vi "Config File Checker v1.2.vi"(8 "Error In":errorcluster) -> (0 "error out":errorcluster, 2 "All Para":cluster{"Auto Para":T1, "General Para 2":T2}={"Auto Para"={"Agitator Delays"=[250, 600], "TF Delays"=[400, 800, 2, 8000], "Insertion Delays"=[100, 400], "Cutting Delays"=[150, 250, 50], "PF Delays"=[300, 8000], "Measur. Delays"=[200.0, 188.9, 1.0], "Reject Delays"=[500], "BF Delays"=[1000, 1000], "P&P Delays"=[1000]}, "General Para 2"={"Max. Cons."=5.0, "Offset 1"=0.0, "Offset 2"=0.0, "Offset 3"=0.0, "Offset 4"=-0.6, "OutputPause"=500.0, "RejectPause"=500.0, "IndexTimeout"=0.0}} {"General Para 2"."Offset 4" format="%.2f"; "General Para 2"."Offset 3" format="%.2f"; "General Para 2"."Offset 2" format="%.2f"; "General Para 2"."Offset 1" format="%.2f"}, 3 "password":string, 5 "file path out":path)   [LabVIEW 2021]
doc: "v1.2:\n- Created new folder if 'data' folder does not exist\n\nV1.1:\n- changed the location of searching and creating the file"
uses:
  RT/Controls/Auto Delays.ctl
  Controls/General Para.ctl
  HMI/Controls/Logging FGV.ctl
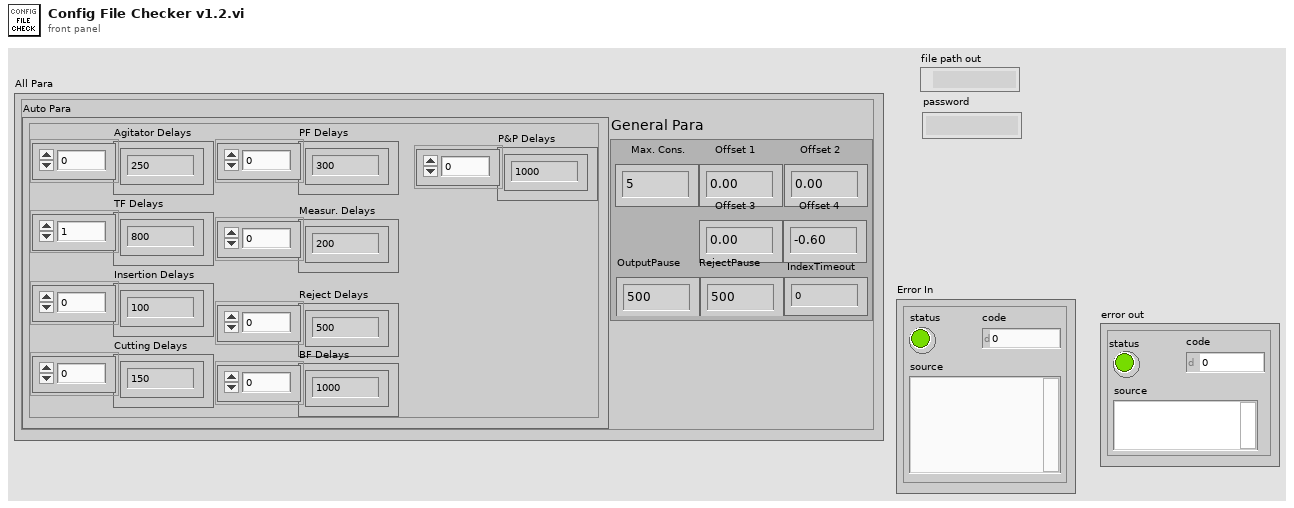
[diagram p1: front panel]
types:
  T1 = typedef "Auto Delays.ctl" = cluster{"Agitator Delays":u32[], "TF Delays":u32[], "Insertion Delays":u32[], "Cutting Delays":u32[], "PF Delays":u32[], "Measur. Delays":dbl[], "Reject Delays":u32[], "BF Delays":u32[], "P&P Delays":u32[]}
  T2 = typedef "General Para.ctl" = cluster{"Max. Cons.":dbl, "Offset 1":dbl, "Offset 2":dbl, "Offset 3":dbl, "Offset 4":dbl, "OutputPause":dbl, "RejectPause":dbl, "IndexTimeout":dbl}
  T3 = typedef "Logging FGV.ctl" = enum16{"Start Shift", "Reload Values", "Log Index", "Read Shift", "Close Shift", "Save Values"}
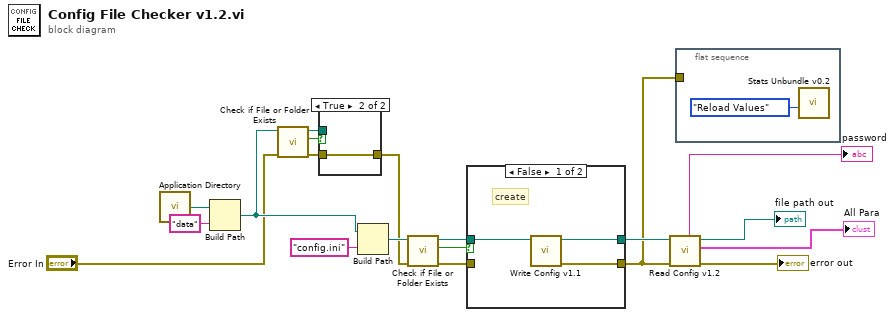
[diagram p0: block diagram]
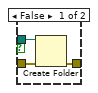
[diagram p2: hidden frame]
diagram:
  n1 = call <vilib>:"Application Directory.vi"() -> ("Application Directory"=w12:path)
  n2 = Build Path(base path=w12, name or relative path="data") -> (appended path=w10:path)
  n3 = call <vilib>:"Check if File or Folder Exists.vi"("error in (no error)"="Error In", "path"=w10) -> ("error out"=w8:errorcluster, "file or folder exists?"=w9:bool, "dup path"=w7:path)  [unwired: 7 in]
  n4 = case shown="True" w9 {
    tunnel: w8 -> [w22 w23]
    tunnel: w7 -> [w21 _]
    tunnel: [w20 w23] -> w5
    frame False {
      n5 = Create Folder(path (use dialog)=w21, error in=w22) -> (error out=w20:errorcluster)  [unwired: 1 in, 2 out]
    }
    frame True {
    }
  }
  n6 = Build Path(base path=w10, name or relative path="config.ini") -> (appended path=w18:path)
  n7 = call <vilib>:"Check if File or Folder Exists.vi"("error in (no error)"=w5, "path"=w18) -> ("error out"=w15:errorcluster, "file or folder exists?"=w17:bool, "dup path"=w16:path)  [unwired: 7 in]
  n8 = case shown="False" w17 {
    tunnel: [w25 w27] -> w14
    tunnel: w16 -> [w26 w27]
    tunnel: w15 -> [_ _]
    tunnel: [w24 _] -> w1
    frame False {
      # "create"
      n9 = call "Write Config v1.1.vi"("file path"=w26) -> ("error out"=w24:errorcluster, "file path out"=w25:path)  [unwired: 9 in]
    }
    frame True {
    }
  }
  n10 = call "Read Config v1.2.vi"("error in"=w1, "file path"=w14) -> ("error out"=→"error out":errorcluster, "All Para"=→"All Para":cluster{"Auto Para":T1, "General Para 2":T2}, "file path out"=→"file path out":path, "password"=→"password":string)  [unwired: 6 in]
  n11 = flat-sequence {
    tunnel: w1 -> [_]
    frame #0 {
      n12 = call "Stats Unbundle v0.2.vi"("State"=Logging_FGV."Reload Values") -> ()  [unwired: 4 in, 7 out]
    }
  }
